vi "FPGA-code.vi"() -> ()   [LabVIEW 2020]
uses:
  <vilib>/Platform/TimedLoop/XDataNode/timing_clust.ctl
  <vilib>/Platform/TimedLoop/XDataNode/nitl_modes.ctl
  <vilib>/Platform/TimedLoop/XDataNode/wakeup.ctl
  <vilib>/rvi/IPIntegrationNode/IPINode_Typedef/niFpgaIPINodeSupportedFamilies.ctl
  <vilib>/rvi/Emulation/niFpgaGetClockAttributes.vi
  <vilib>/rvi/Emulation/niFpgaSctlEmulationGetInTimedLoop.vi
  <vilib>/rvi/Emulation/niFpgaEmulationReportErrorSimple.vi
  <vilib>/rvi/eio/common/nirviEmuTemplateMethod_errors.vi
  <vilib>/rvi/interface/RandomDataEmulation/nirviRandomDataMultiElementFPGAFIFO.vi
  <instcachedir>/0/nirviRandomDataMultiElementFPGAFIFO_3E9965BA1FAD4E7B8DABA31768A09B1F.lvgen/nirviRandomDataMultiElementFPGAFIFO_3E9965BA1FAD4E7B8DABA31768A09B1F_001.vi
  <vilib>/rvi/interface/RandomDataEmulation/niFpgaRandomDataHandleErrors.vi
  <vilib>/rvi/Emulation/niFpgaCriticalErrorInLSC.vi
  <instcachedir>/0/nirviRandomDataMultiElementFPGAFIFO_3E9965BA1FAD4E7B8DABA31768A09B1F.lvgen/nirviRandomDataMultiElementFPGAFIFO_3E9965BA1FAD4E7B8DABA31768A09B1F_000.vi
  <vilib>/rvi/IPIntegrationNode/IPINode_Utilities/niFpgaIPINodeSimCore.vi
  <vilib>/eio/EIONode/EIONode.xnode
  <vilib>/rvi/DataTransferAndStorage/Container/XNode/niFpgaContainer.xnode
  <vilib>/rvi/interface/RandomDataEmulation/nirviRandomDataFpgaMultiElementTemplate.vi
  <vilib>/rvi/interface/RandomDataEmulation/nirviRandomDataFpgaReadWriteTemplate.vi
  <vilib>/platform/TimedLoop/XDataNode/XDataNode.xnode
  <vilib>/rvi/IPIntegrationNode/IPINode_Xnode/niFpgaIPINode.xnode
  Simulink_ANN/hdl_prj/hdlsrc/ANN/IP_BlockSimFiles/xsim.dir/HDL_ANN/xsimk430938EFC64F42458762135EEBE48214.dll
  <vilib>/rvi/Memory/Memory_Emulation/nirvimemoryFastEmulation.vi
  <vilib>/rvi/Memory/Memory_Emulation/nirvimemoryEmulation.vi
  Global var FPGA.vi
  <vilib>/rvi/FIFO/Fifo_Resource/niFpgaFifoEmulationRefIn.vi
  <vilib>/Platform/TimedLoop/XDataNode/XDNodeRunTimeDep.lvlib
panel:
  out "Training Done":bool
  out "Inputs":bool[](array[boolean])
  out "Updated Weights and Biases":sgl[](array[numeric])
  out "2ndHiddenOut":sgl[](array[numeric])
  out "hidden 1":sgl[](array[numeric])
  out "Numeric":i32
  out "Data Read on iteration":i32
  out "Loop iteration":i32
  out "#Windows Handled":i16
  out "OutputLayerOut":sgl
  in  "Learning Rate":sgl=0.01
  in  "Data inputs":sgl=8.0
  out "Label expected output":sgl
  out "Initial Weigths and Biases":sgl[](array[numeric]) format="%.2f"
  out "Case Sleector":i16=3
  in  "stop":bool
  out "Array recived to multiply":sgl[](array[numeric])
  out "input Timed Out?":bool
  # "Node Values"
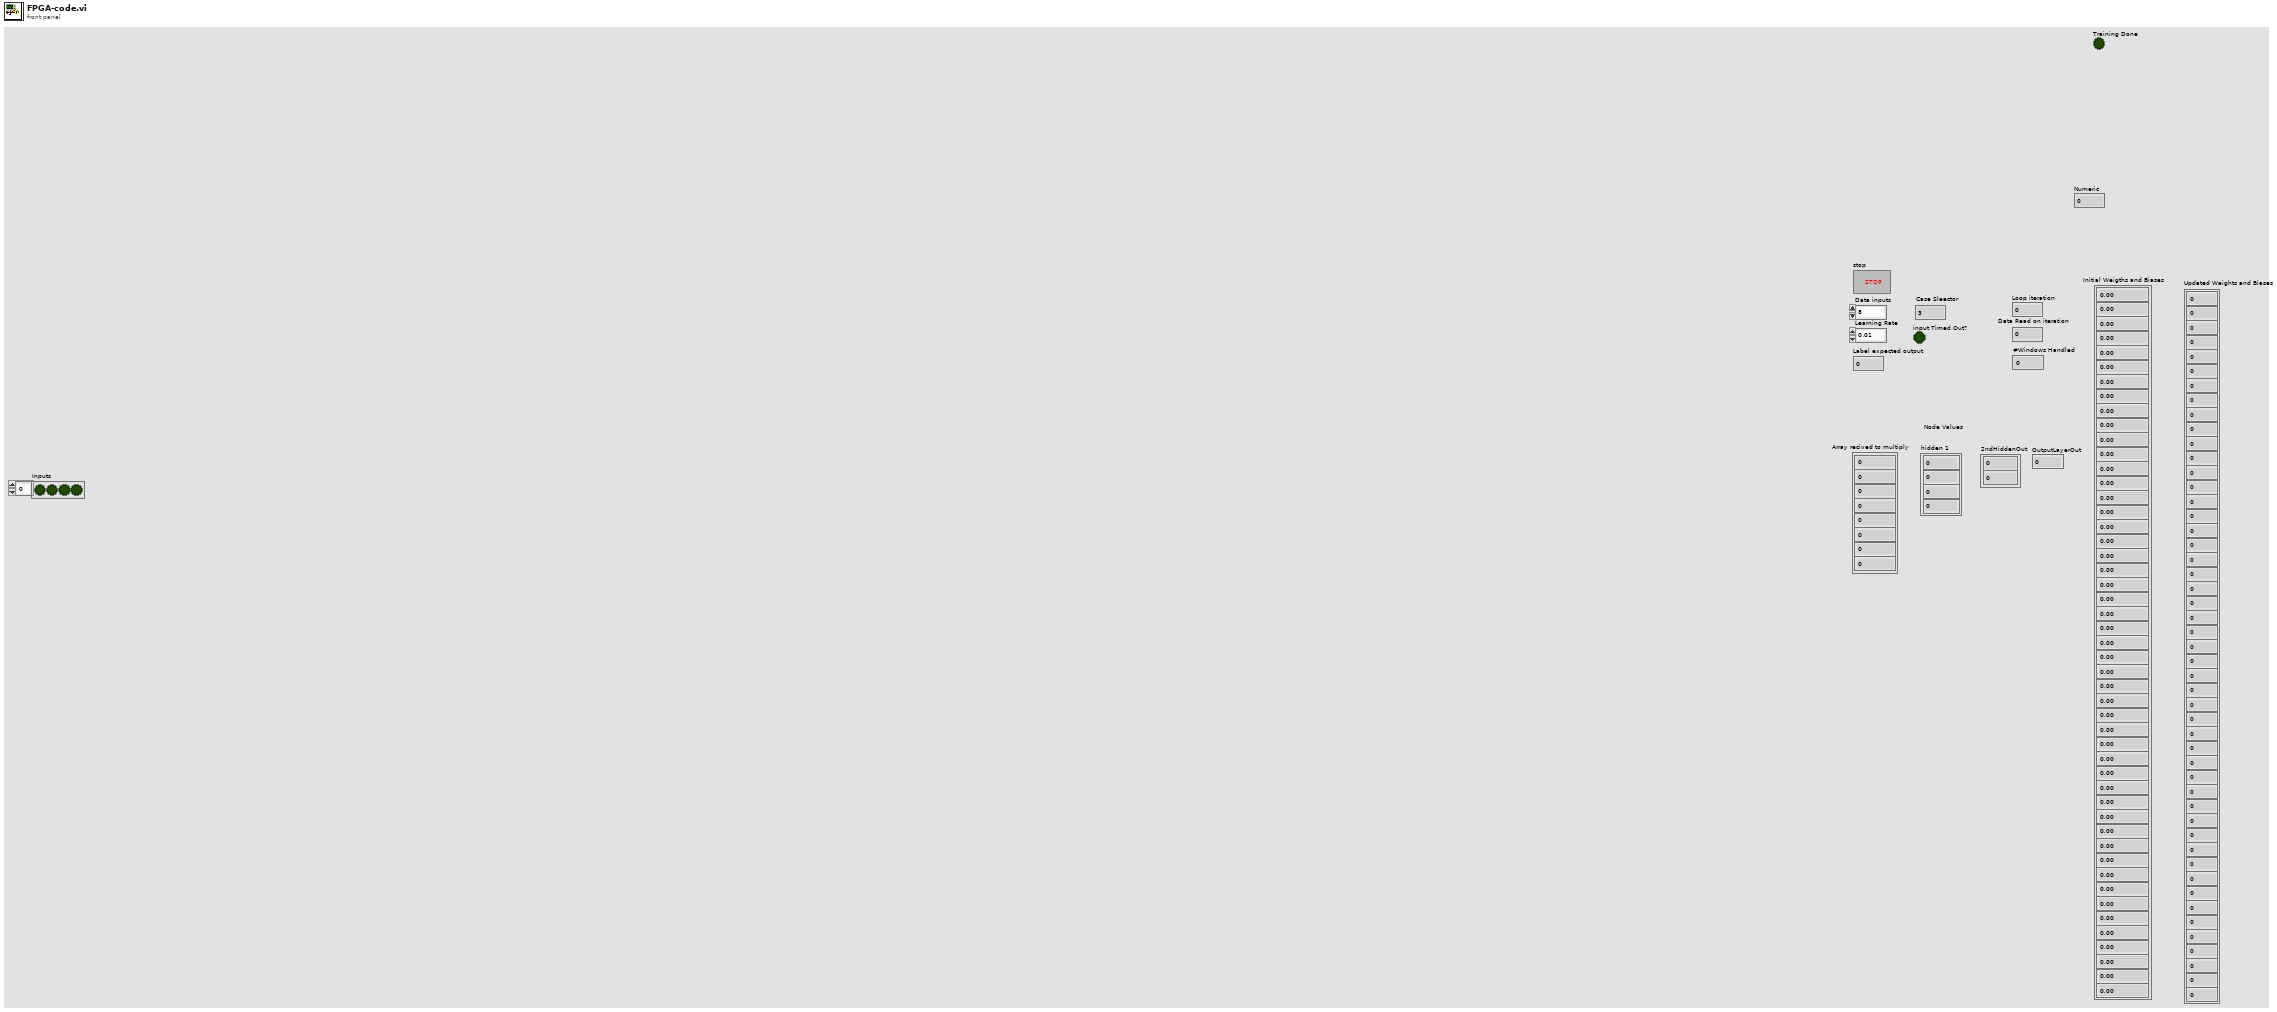
[diagram p1: front panel]
types:
  T1 = typedef "niFpgaIPINodeSupportedFamilies.ctl" = cluster{"unlimited?":bool, "supported targets":string[]}
  T2 = typedef "XDNodeRunTimeDep.lvlib/timing_clust.ctl" = cluster{"Expected End [f-1]":u64, "Actual End [f-1]":u64, "Finished Late? [f-1]":bool, "Expected End [i-1]":u64, "Actual End [i-1]":u64, "Finished Late? [i-1]":bool, "Expected Start [i]":u64, "Actual Start [i]":u64, "Expected Start [f]":u64, "Actual Start [f]":u64, "Source Name":string, "Structure Name":string, "Period":i64, "Deadline":i64, "Offset":i64, "Start":i64, "Priority":i32, "Timeout":i32, "Mode":T3, "Wakeup Reason":T4, "Error":errorcluster, "Source Type":string, "Secondary Source Type":string, "Global End Time":u64, "Global Start Time":u64, "Frame Duration":u64, "Iteration Duration":u64, "Assigned CPU":i32, "I/O Scan Engine Mode":u32}
  T3 = typedef "XDNodeRunTimeDep.lvlib/nitl_modes.ctl" = enum32{"No Change", "Process missed periods, maintain original phase", "Discard missed periods, maintain original phase", "Process missed periods, ignore original phase", "Discard missed periods, ignore original phase"}
  T4 = typedef "XDNodeRunTimeDep.lvlib/wakeup.ctl" = enum32{"Normal", "Aborted", "Asynchronous wakeup", "Timing source error", "Timed loop error", "Timeout"}
  T5 = cluster{"[0]":sgl, "[1]":sgl, "[2]":sgl, "[3]":sgl, "[4]":sgl, "[5]":sgl, "[6]":sgl, "[7]":sgl, "[8]":sgl, "[9]":sgl, "[10]":sgl, "[11]":sgl, "[12]":sgl, "[13]":sgl, "[14]":sgl, "[15]":sgl, "[16]":sgl, "[17]":sgl, "[18]":sgl, "[19]":sgl, "[20]":sgl, "[21]":sgl, "[22]":sgl, "[23]":sgl, "[24]":sgl}
  T6 = cluster{"Element[0]":sgl, "Element[1]":sgl, "Element[2]":sgl}
  T7 = cluster{sgl, sgl, sgl, sgl, sgl, sgl, sgl, sgl, sgl, sgl, sgl, sgl, sgl, sgl, sgl, sgl, sgl, sgl, sgl, sgl, sgl, sgl, sgl, sgl, sgl}
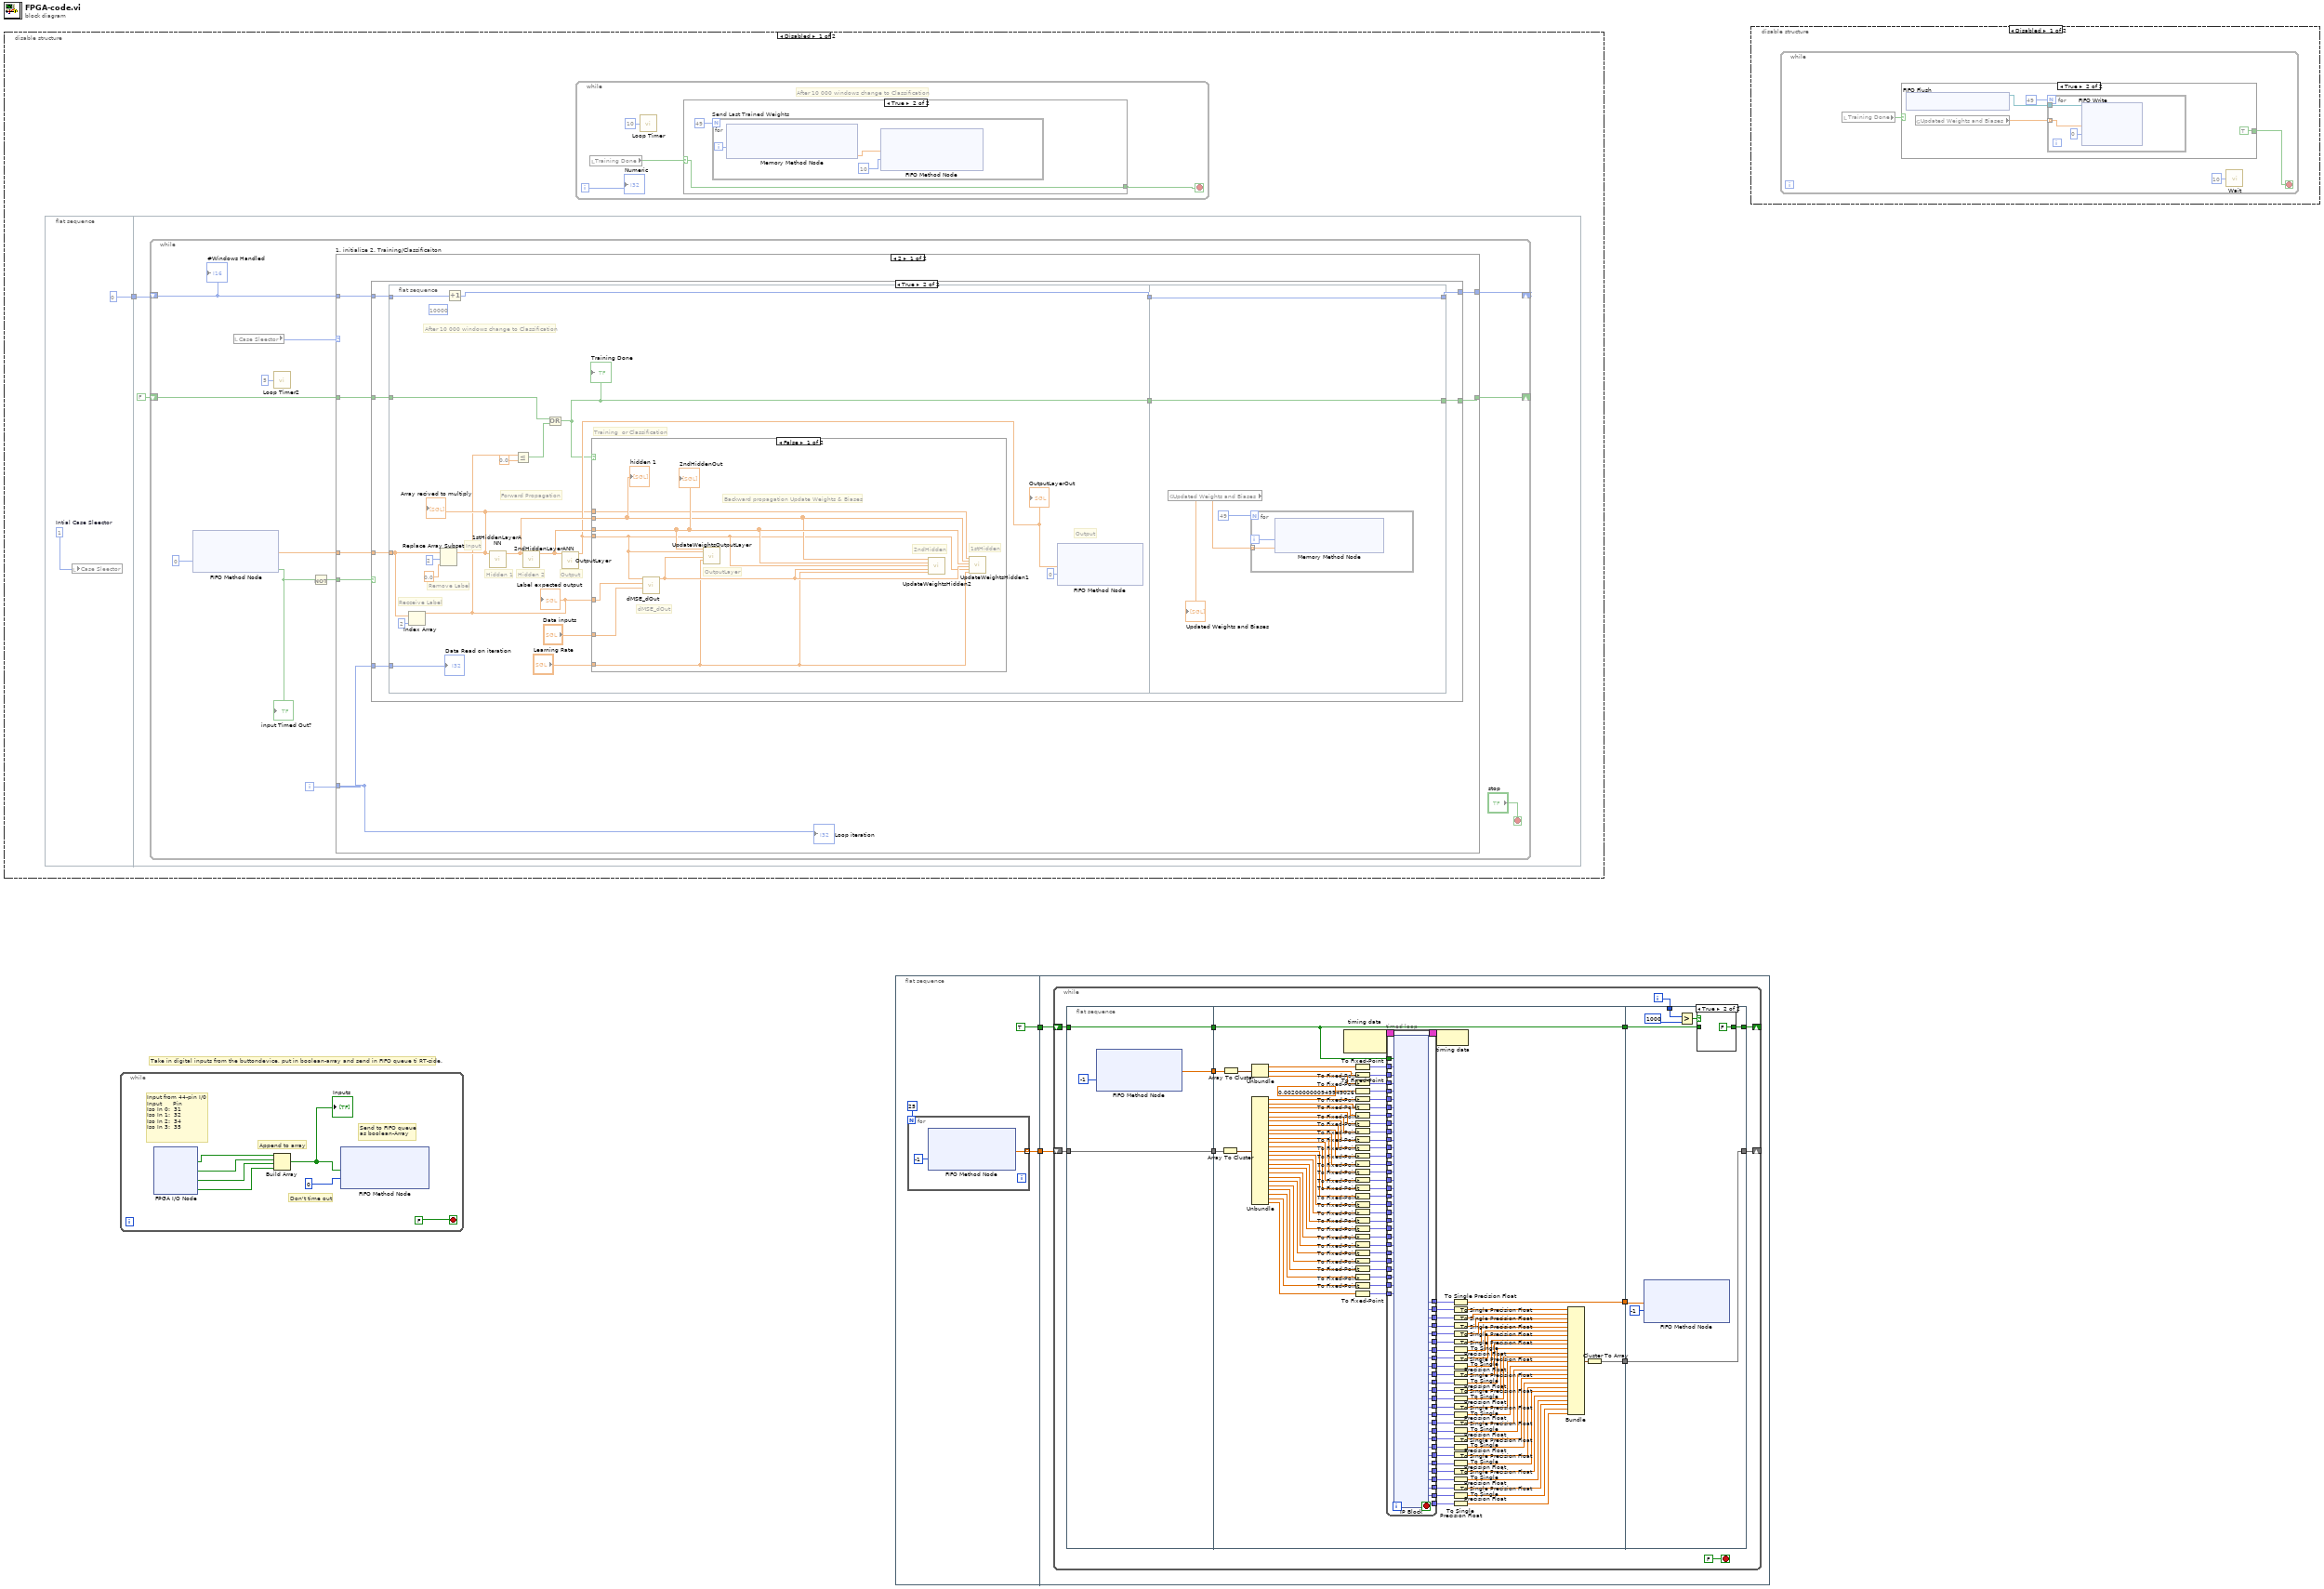
[diagram p0: block diagram]
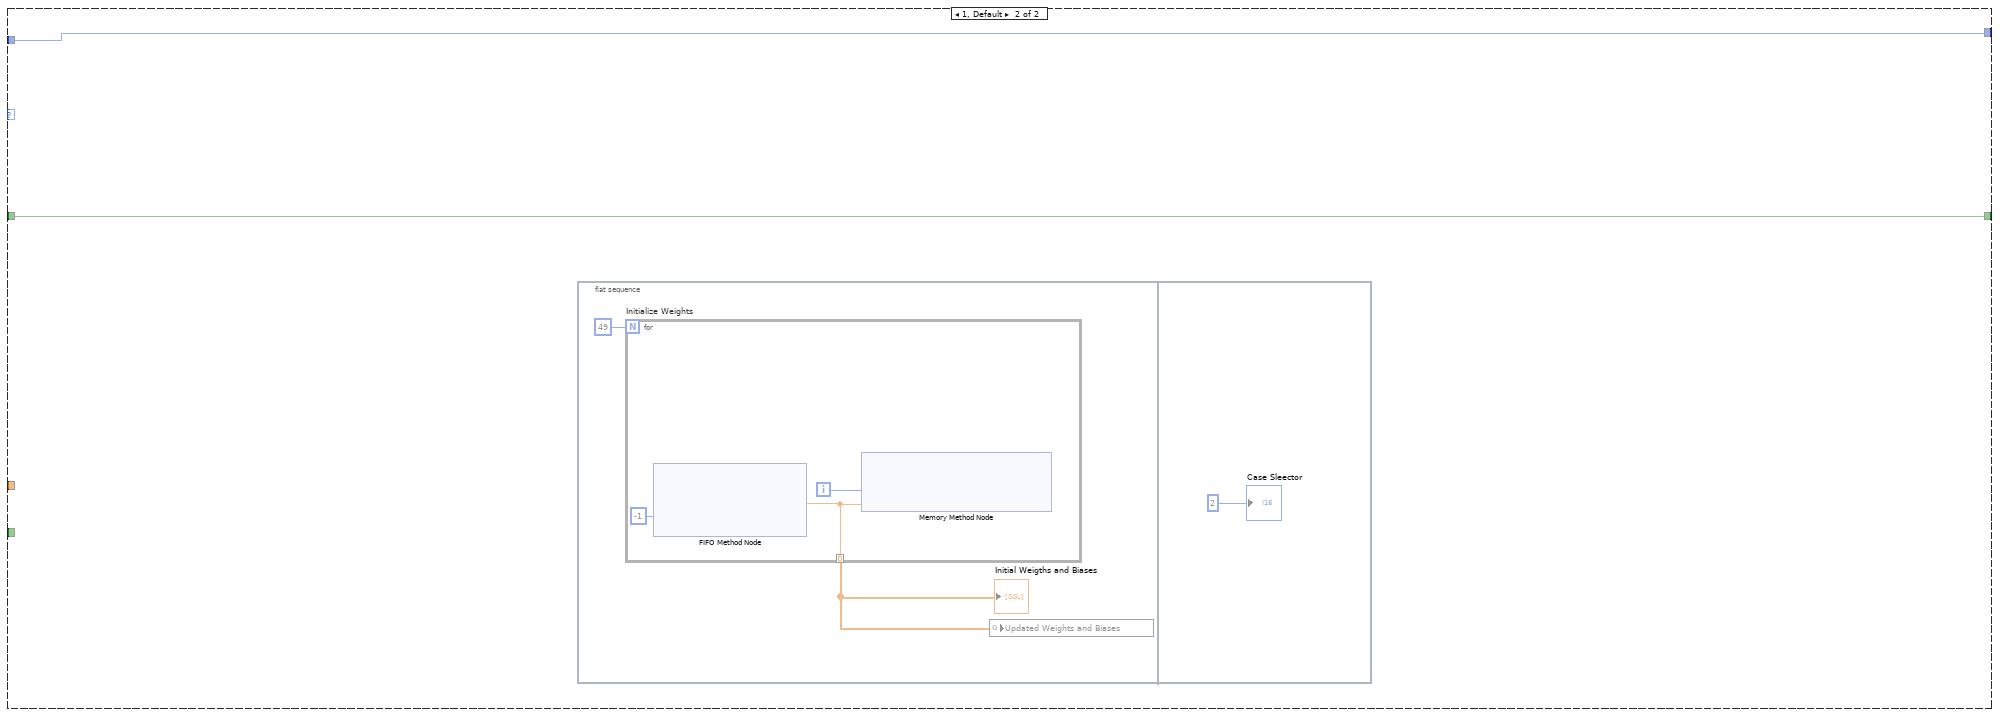
[diagram p5: hidden frame]
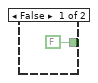
[diagram p8: hidden frame]
diagram:
  # "Take in digital inputs from the buttondevice, put in boolean-array and send in FIFO queue ti RT-side."
  n1 = disable-structure shown="Disabled" {
    frame Disabled {
      n2 = flat-sequence {
        tunnel: [i16 0] -> w3
        tunnel: w3 -> [w17]
        frame #0 {
          w15 = i16 1  # Intial Case Sleector
          n3 = local write "Case Sleector"(w15) -> ()
        }
        frame #1 {
          n4 = while {
            shift-right: [w24] -> _
            shift-left: w17 -> [w23]
            shift-right: [w18] -> _
            shift-left: FALSE -> [w19]
            i -> [w27]
            stop <- "stop" stop-if-true
            n5 = xnode ("FIFO Method Node")("Timeout"=0) -> ("Element"=w22:sgl[], "Timed Out?"=w26:bool)  [unwired: 2 in, 2 out]
            "input Timed Out?" <- w26
            n6 = local read "Case Sleector"() -> (w29:i16)
            n7 = call "Loop Timer2"("Count(mSec)"=u32 5) -> ()  [unwired: 1 out]
            n8 = Not(x=w26) -> (.not. x?=w25:bool)
            n9 = case "1. initialize 2. Training/Classificaiton" shown="2" w29 {
              tunnel: w27 -> [w35 _]
              tunnel: w25 -> [w36 _]
              tunnel: w23 -> [w34 w81]
              tunnel: [w33 w81] -> w24
              tunnel: w22 -> [w32 _]
              tunnel: w19 -> [w31 w80]
              tunnel: [w30 w80] -> w18
              frame 2 {
                n10 = case shown="True" w36 {
                  tunnel: w35 -> [_ w46]
                  tunnel: w34 -> [w38 w45]
                  tunnel: [w38 w44] -> w33
                  tunnel: w32 -> [_ w43]
                  tunnel: w31 -> [w37 w41]
                  tunnel: [w37 w39] -> w30
                  frame False {
                  }
                  frame True {
                    n11 = flat-sequence {
                      tunnel: w46 -> [w65]
                      tunnel: w45 -> [w64]
                      tunnel: w43 -> [w55]
                      tunnel: [w63] -> w42
                      tunnel: w41 -> [w47]
                      tunnel: [w49] -> w40
                      tunnel: [w77] -> w44
                      tunnel: w42 -> [w77]
                      tunnel: w40 -> [w75]
                      tunnel: [w75] -> w39
                      frame #0 {
                        (unwired) i16 10000 ("y")
                        # "Recceive Label"
                        # "Remove Label"
                        # "Training  or Classification"
                        # "After 10 000 windows change to Classification"
                        # "Output"
                        # "Output"
                        # "Hidden 2"
                        # "Hidden 1"
                        # "Input"
                        # "Forward Propagation"
                        n12 = Index Array(array=w55, index=2) -> (element=w51:sgl)
                        "Label expected output" <- w51
                        n13 = Replace Array Subset(array=w55, new element=sgl 0.0 ("new element/subarray"), index=2) -> (w53:sgl[])
                        "Array recived to multiply" <- w53
                        n14 = Increment(x=w64) -> (x+1=w63:i16)
                        n15 = call "1stHiddenLayerANN.vi"("Input"=w53) -> ("1stHiddenOut"=w61:sgl[])  [unwired: 10 in]
                        n16 = Less Or Equal?(x=w51, y=sgl 0.0) -> (x <= y?=w48:bool)
                        n17 = call "2ndHiddenLayerANN.vi"("2nd HiddenIn"=w61) -> ("2ndHiddenOut"=w59:sgl[])  [unwired: 9 in]
                        n18 = Or(x=w47, y=w48) -> (x .or. y?=w49:bool)
                        "Training Done" <- w49
                        n19 = call "OutputLayer.vi"("OutputlayerIn"=w59) -> ("OutputLayerOut"=w58:sgl)  [unwired: 14 in]
                        "OutputLayerOut" <- w58
                        n20 = case shown="False" w49 {
                          tunnel: "Data inputs" -> [w67 _]
                          tunnel: w61 -> [w70 _]
                          tunnel: "Learning Rate" -> [w72 _]
                          tunnel: w58 -> [w69 _]
                          tunnel: w59 -> [w71 _]
                          tunnel: w51 -> [w68 _]
                          tunnel: w53 -> [w66 _]
                          frame False {
                            # "1stHidden"
                            # "2ndHidden"
                            # "OutputLayer"
                            # "dMSE_dOut"
                            # "Backward propagation Update Weights & Biases"
                            n21 = call "dMSE_dOut.vi"("Data inputs"=w67, "Label (expected output"=w68, "Output"=w69) -> ("Numeric"=w73:sgl)  [unwired: 8 in]
                            n22 = call "UpdateWeightsOutputLayer.vi"("OutputH2"=w71, "Final Output"=w69, "dEtot_dOut"=w73, "Learning Rate"=w72) -> ()  [unwired: 16 in]
                            n23 = call "UpdateWeightsHidden2.vi"("OutH1"=w70, "OutH2"=w71, "Output"=w69, "dEtot_dOut"=w73, "Learning Rate"=w72) -> ()  [unwired: 11 in]
                            n24 = call "UpdateWeightsHidden1.vi"("Input"=w66, "OutH1"=w70, "OutH2"=w71, "dEOut_dOut"=w73, "Output"=w69, "Learning Rate"=w72) -> ()  [unwired: 14 in]
                            "hidden 1" <- w70
                            "2ndHiddenOut" <- w71
                          }
                          frame True {
                          }
                        }
                        n25 = xnode ("FIFO Method Node")("Element"=w58, "Timeout"=0) -> ()  [unwired: 1 in, 2 out]
                        "Data Read on iteration" <- w65
                      }
                      frame #1 {
                        n26 = global read "Global var FPGA.vi" "Updated Weights and Biases"() -> (w76:sgl[])
                        "Updated Weights and Biases" <- w76
                        n27 = for "Send Last Trained Weights" {
                          N: 49 -> [_]
                          tunnel: w76 -> [w78] mode=indexing
                          i -> [w79]
                          n28 = xnode ("Memory Method Node")("Address"=w79, "Data"=w78) -> ()  [unwired: 1 in, 1 out]
                        }
                      }
                    }
                  }
                }
                "Loop iteration" <- w35
              }
              frame 1, Default {
                n29 = flat-sequence {
                  frame #0 {
                    n30 = for "Initialize Weights" {
                      N: 49 -> [_]
                      tunnel: [w84] -> w82 mode=indexing
                      i -> [w86]
                      n31 = xnode ("FIFO Method Node")("Timeout"=-1) -> ("Element"=w84:sgl)  [unwired: 1 in, 2 out]
                      n32 = xnode ("Memory Method Node")("Address"=w86, "Data"=w84) -> ()  [unwired: 1 in, 1 out]
                    }
                    "Initial Weigths and Biases" <- w82
                    n33 = global write "Global var FPGA.vi" "Updated Weights and Biases"(w82) -> ()
                  }
                  frame #1 {
                    "Case Sleector" <- i16 2 ("Numeric 3")
                  }
                }
              }
            }
            "#Windows Handled" <- w23
          }
        }
      }
      n34 = while {
        i -> [w5]
        stop <- w6 stop-if-true
        # "After 10 000 windows change to Classification"
        n35 = local read "Training Done"() -> (w7:bool)
        n36 = call "Loop Timer"("Count(mSec)"=u32 10) -> ()  [unwired: 1 out]
        n37 = case shown="True" w7 {
          selector: w7 -> [w8 w9]
          tunnel: [w8 w9] -> w6
          frame False {
          }
          frame True {
            n38 = for "Send Last Trained Weights" {
              N: 49 -> [_]
              i -> [w13]
              n39 = xnode ("Memory Method Node")("Address"=w13) -> ("Data"=w12:sgl)  [unwired: 1 in, 1 out]
              n40 = xnode ("FIFO Method Node")("Element"=w12, "Timeout"=10) -> ()  [unwired: 1 in, 2 out]
            }
          }
        }
        "Numeric" <- w5
      }
    }
    frame Enabled {
    }
  }
  n41 = while {
    stop <- FALSE stop-if-true
    # "Don't time out"
    # "Append to array"
    # "Send to FIFO queue\nas boolean-Array"
    # "Input from 44-pin I/0\nInput      Pin\nIso In 0:  31\nIso In 1:  32\nIso In 2:  34\nIso In 3:  35"
    n42 = xnode "FPGA I/O Node"() -> ("Iso In 0"=w93:bool, "Iso In 1"=w90:bool, "Iso In 2"=w89:bool, "Iso In 3"=w88:bool)  [unwired: 4 in, 4 out]
    n43 = Build Array(w93, w90, w89, w88) -> (w91:bool[])
    "Inputs" <- w91
    n44 = xnode ("FIFO Method Node")("Element"=w91, "Timeout"=0) -> ()  [unwired: 1 in, 2 out]
  }
  n45 = flat-sequence {
    tunnel: [w96] -> w2
    tunnel: [TRUE] -> w1
    tunnel: w2 -> [w101]
    tunnel: w1 -> [w100]
    frame #0 {
      n46 = for {
        N: 25 -> [_]
        tunnel: [w98] -> w96 mode=indexing
        n47 = xnode ("FIFO Method Node")("Timeout"=-1) -> ("Element"=w98:sgl)  [unwired: 1 in, 2 out]
      }
    }
    frame #1 {
      n48 = while {
        shift-right: [w109] -> _
        shift-left: w101 -> [w108]
        shift-right: [w106] -> _
        shift-left: w100 -> [w103]
        i -> [w102]
        stop <- FALSE stop-if-true
        n49 = flat-sequence {
          tunnel: [w115] -> w113
          tunnel: [w116] -> w112
          tunnel: w108 -> [w115]
          tunnel: [w114] -> w104
          tunnel: w103 -> [w114]
          tunnel: w113 -> [w130]
          tunnel: w112 -> [w212]
          tunnel: [w127] -> w110
          tunnel: [w125] -> w107
          tunnel: [w120] -> w105
          tunnel: w104 -> [w120]
          tunnel: w110 -> [w561]
          tunnel: [w561] -> w109
          tunnel: w107 -> [w560]
          tunnel: [w559] -> w106
          tunnel: w105 -> [w558]
          tunnel: w102 -> [w556]
          frame #0 {
            n50 = xnode ("FIFO Method Node")("Timeout"=-1) -> ("Element"=w116:sgl[])  [unwired: 2 in, 3 out]
          }
          frame #1 {
            n51 = Array To Cluster(array=w130) -> (cluster=w180:T5)
            n52 = Array To Cluster(array=w212) -> (cluster=w211:T6)
            n53 = Unbundle(w211) -> ("Element[0]"=w210:sgl, "Element[1]"=w209:sgl, "Element[2]"=w123:sgl)
            n54 = Unbundle(w180) -> ("[0]"=w208:sgl, "[1]"=w236:sgl, "[2]"=w235:sgl, "[3]"=w234:sgl, "[4]"=w233:sgl, "[5]"=w232:sgl, "[6]"=w231:sgl, "[7]"=w230:sgl, "[8]"=w229:sgl, "[9]"=w228:sgl, "[10]"=w227:sgl, "[11]"=w226:sgl, "[12]"=w225:sgl, "[13]"=w224:sgl, "[14]"=w223:sgl, "[15]"=w222:sgl, "[16]"=w221:sgl, "[17]"=w220:sgl, "[18]"=w219:sgl, "[19]"=w218:sgl, "[20]"=w217:sgl, "[21]"=w216:sgl, "[22]"=w215:sgl, "[23]"=w214:sgl, "[24]"=w213:sgl)
            n55 = node-c288() -> (w119:T2)  [unwired: 1 in]
            n56 = To Fixed-Point(number=w210) -> (fixed-point=w207:fxp<+/-,18,12>)  [unwired: 1 in]
            n57 = To Fixed-Point(number=w209) -> (fixed-point=w206:fxp<+/-,18,12>)  [unwired: 1 in]
            n58 = To Fixed-Point(number=w123) -> (fixed-point=w124:fxp<+/-,18,12>)  [unwired: 1 in]
            n59 = To Fixed-Point(number=sgl 0.002) -> (fixed-point=w122:fxp<+/-,18,12>)  [unwired: 1 in]
            n60 = To Fixed-Point(number=w208) -> (fixed-point=w205:fxp<+/-,18,12>)  [unwired: 1 in]
            n61 = To Fixed-Point(number=w236) -> (fixed-point=w204:fxp<+/-,18,12>)  [unwired: 1 in]
            n62 = To Fixed-Point(number=w235) -> (fixed-point=w203:fxp<+/-,18,12>)  [unwired: 1 in]
            n63 = To Fixed-Point(number=w234) -> (fixed-point=w202:fxp<+/-,18,12>)  [unwired: 1 in]
            n64 = To Fixed-Point(number=w233) -> (fixed-point=w201:fxp<+/-,18,12>)  [unwired: 1 in]
            n65 = To Fixed-Point(number=w232) -> (fixed-point=w200:fxp<+/-,18,12>)  [unwired: 1 in]
            n66 = To Fixed-Point(number=w231) -> (fixed-point=w199:fxp<+/-,18,12>)  [unwired: 1 in]
            n67 = To Fixed-Point(number=w230) -> (fixed-point=w198:fxp<+/-,18,12>)  [unwired: 1 in]
            n68 = To Fixed-Point(number=w229) -> (fixed-point=w197:fxp<+/-,18,12>)  [unwired: 1 in]
            n69 = To Fixed-Point(number=w228) -> (fixed-point=w196:fxp<+/-,18,12>)  [unwired: 1 in]
            n70 = To Fixed-Point(number=w227) -> (fixed-point=w195:fxp<+/-,18,12>)  [unwired: 1 in]
            n71 = To Fixed-Point(number=w226) -> (fixed-point=w194:fxp<+/-,18,12>)  [unwired: 1 in]
            n72 = To Fixed-Point(number=w225) -> (fixed-point=w193:fxp<+/-,18,12>)  [unwired: 1 in]
            n73 = To Fixed-Point(number=w224) -> (fixed-point=w192:fxp<+/-,18,12>)  [unwired: 1 in]
            n74 = To Fixed-Point(number=w223) -> (fixed-point=w191:fxp<+/-,18,12>)  [unwired: 1 in]
            n75 = To Fixed-Point(number=w222) -> (fixed-point=w190:fxp<+/-,18,12>)  [unwired: 1 in]
            n76 = To Fixed-Point(number=w221) -> (fixed-point=w189:fxp<+/-,18,12>)  [unwired: 1 in]
            n77 = To Fixed-Point(number=w220) -> (fixed-point=w188:fxp<+/-,18,12>)  [unwired: 1 in]
            n78 = To Fixed-Point(number=w219) -> (fixed-point=w187:fxp<+/-,18,12>)  [unwired: 1 in]
            n79 = To Fixed-Point(number=w218) -> (fixed-point=w186:fxp<+/-,18,12>)  [unwired: 1 in]
            n80 = To Fixed-Point(number=w217) -> (fixed-point=w185:fxp<+/-,18,12>)  [unwired: 1 in]
            n81 = To Fixed-Point(number=w216) -> (fixed-point=w184:fxp<+/-,18,12>)  [unwired: 1 in]
            n82 = To Fixed-Point(number=w215) -> (fixed-point=w183:fxp<+/-,18,12>)  [unwired: 1 in]
            n83 = To Fixed-Point(number=w214) -> (fixed-point=w182:fxp<+/-,18,12>)  [unwired: 1 in]
            n84 = To Fixed-Point(number=w213) -> (fixed-point=w181:fxp<+/-,18,12>)  [unwired: 1 in]
            n85 = timed-loop {
              timing: w119 -> [_]
              timing-out: [_] -> w118
              tunnel: w207 -> [w292]
              tunnel: w206 -> [w291]
              tunnel: w205 -> [w290]
              tunnel: w204 -> [w289]
              tunnel: w203 -> [w288]
              tunnel: w202 -> [w287]
              tunnel: w201 -> [w286]
              tunnel: w200 -> [w285]
              tunnel: w199 -> [w284]
              tunnel: w198 -> [w283]
              tunnel: w197 -> [w282]
              tunnel: w196 -> [w281]
              tunnel: w195 -> [w280]
              tunnel: w194 -> [w279]
              tunnel: w193 -> [w278]
              tunnel: w192 -> [w277]
              tunnel: w191 -> [w276]
              tunnel: w190 -> [w275]
              tunnel: w189 -> [w274]
              tunnel: w188 -> [w273]
              tunnel: w187 -> [w272]
              tunnel: w186 -> [w271]
              tunnel: w185 -> [w270]
              tunnel: w184 -> [w269]
              tunnel: w183 -> [w268]
              tunnel: w182 -> [w267]
              tunnel: w181 -> [w266]
              tunnel: [w265] -> w179
              tunnel: [w264] -> w178
              tunnel: [w263] -> w177
              tunnel: [w262] -> w176
              tunnel: [w261] -> w175
              tunnel: [w260] -> w174
              tunnel: [w259] -> w173
              tunnel: [w258] -> w172
              tunnel: [w257] -> w171
              tunnel: [w256] -> w170
              tunnel: [w255] -> w169
              tunnel: [w254] -> w168
              tunnel: [w253] -> w167
              tunnel: [w252] -> w166
              tunnel: [w251] -> w165
              tunnel: [w250] -> w164
              tunnel: [w249] -> w163
              tunnel: [w248] -> w162
              tunnel: [w247] -> w161
              tunnel: [w246] -> w160
              tunnel: [w245] -> w159
              tunnel: [w244] -> w158
              tunnel: [w243] -> w157
              tunnel: [w242] -> w156
              tunnel: [w241] -> w147
              tunnel: [w240] -> w126
              tunnel: w124 -> [w239]
              tunnel: w122 -> [w238]
              tunnel: w120 -> [w237]
              stop <- _ stop-if-true
              n86 = xnode ("IP Block")("train_1"=w237, "input_0"=w292, "input_1"=w291, "target"=w239, "alpha"=w238, "w1_0"=w290, "w1_1"=w289, "w1_2"=w288, "w1_3"=w287, "w1_4"=w286, "w1_5"=w285, "w1_6"=w284, "w1_7"=w283, "w2_0"=w282, "w2_1"=w281, "w2_2"=w280, "w2_3"=w279, "w2_4"=w278, "w2_5"=w277, "w2_6"=w276, "w2_7"=w275, "w3_0"=w274, "w3_1"=w273, "b1_0"=w272, "b1_1"=w271, "b1_2"=w270, "b1_3"=w269, "b2_0"=w268, "b2_1"=w267, "b3"=w266) -> ("output"=w240:fxp<+/-,18,12>, "w1_out_0"=w265:fxp<+/-,18,12>, "w1_out_1"=w263:fxp<+/-,18,12>, "w1_out_2"=w262:fxp<+/-,18,12>, "w1_out_3"=w261:fxp<+/-,18,12>, "w1_out_4"=w260:fxp<+/-,18,12>, "w1_out_5"=w259:fxp<+/-,18,12>, "w1_out_6"=w258:fxp<+/-,18,12>, "w1_out_7"=w257:fxp<+/-,18,12>, "w2_out_0"=w256:fxp<+/-,18,12>, "w2_out_1"=w250:fxp<+/-,18,12>, "w2_out_2"=w251:fxp<+/-,18,12>, "w2_out_3"=w252:fxp<+/-,18,12>, "w2_out_4"=w253:fxp<+/-,18,12>, "w2_out_5"=w249:fxp<+/-,18,12>, "w2_out_6"=w248:fxp<+/-,18,12>, "w2_out_7"=w247:fxp<+/-,18,12>, "w3_out_0"=w254:fxp<+/-,18,12>, "w3_out_1"=w246:fxp<+/-,18,12>, "b1_out_0"=w245:fxp<+/-,18,12>, "b1_out_1"=w244:fxp<+/-,18,12>, "b1_out_2"=w243:fxp<+/-,18,12>, "b1_out_3"=w242:fxp<+/-,18,12>, "b2_out_0"=w255:fxp<+/-,18,12>, "b2_out_1"=w264:fxp<+/-,18,12>, "b3_out"=w241:fxp<+/-,18,12>)
            }
            n87 = node-c288(w118) -> ()
            n88 = To Single Precision Float(number=w126) -> (single precision float=w125:sgl)
            n89 = To Single Precision Float(number=w179) -> (single precision float=w129:sgl)
            n90 = To Single Precision Float(number=w177) -> (single precision float=w155:sgl)
            n91 = To Single Precision Float(number=w176) -> (single precision float=w154:sgl)
            n92 = To Single Precision Float(number=w175) -> (single precision float=w153:sgl)
            n93 = To Single Precision Float(number=w174) -> (single precision float=w152:sgl)
            n94 = To Single Precision Float(number=w173) -> (single precision float=w151:sgl)
            n95 = To Single Precision Float(number=w172) -> (single precision float=w150:sgl)
            n96 = To Single Precision Float(number=w171) -> (single precision float=w149:sgl)
            n97 = To Single Precision Float(number=w170) -> (single precision float=w148:sgl)
            n98 = To Single Precision Float(number=w164) -> (single precision float=w146:sgl)
            n99 = To Single Precision Float(number=w165) -> (single precision float=w145:sgl)
            n100 = To Single Precision Float(number=w166) -> (single precision float=w144:sgl)
            n101 = To Single Precision Float(number=w167) -> (single precision float=w143:sgl)
            n102 = To Single Precision Float(number=w163) -> (single precision float=w142:sgl)
            n103 = To Single Precision Float(number=w162) -> (single precision float=w141:sgl)
            n104 = To Single Precision Float(number=w161) -> (single precision float=w140:sgl)
            n105 = To Single Precision Float(number=w168) -> (single precision float=w139:sgl)
            n106 = To Single Precision Float(number=w160) -> (single precision float=w138:sgl)
            n107 = To Single Precision Float(number=w159) -> (single precision float=w137:sgl)
            n108 = To Single Precision Float(number=w158) -> (single precision float=w136:sgl)
            n109 = To Single Precision Float(number=w157) -> (single precision float=w135:sgl)
            n110 = To Single Precision Float(number=w156) -> (single precision float=w134:sgl)
            n111 = To Single Precision Float(number=w169) -> (single precision float=w133:sgl)
            n112 = To Single Precision Float(number=w178) -> (single precision float=w132:sgl)
            n113 = To Single Precision Float(number=w147) -> (single precision float=w131:sgl)
            n114 = Bundle(w129, w155, w154, w153, w152, w151, w150, w149, w148, w146, w145, w144, w143, w142, w141, w140, w139, w138, w137, w136, w135, w134, w133, w132, w131) -> (w128:T7)  [unwired: 1 in]
            n115 = Cluster To Array(cluster=w128) -> (array=w127:sgl[])
          }
          frame #2 {
            n116 = xnode ("FIFO Method Node")("Element"=w560, "Timeout"=-1) -> ()  [unwired: 1 in, 2 out]
            n117 = Greater?(x=w556, y=i16 1000) -> (0:w555:bool)
            n118 = case shown="True" w555 {
              tunnel: [w562 FALSE] -> w559
              tunnel: w558 -> [w562 _]
              frame False {
              }
              frame True {
              }
            }
          }
        }
      }
    }
  }
  n119 = disable-structure shown="Disabled" {
    frame Disabled {
      n120 = while {
        stop <- w564 stop-if-true
        n121 = local read "Training Done"() -> (w565:bool)
        n122 = case shown="True" w565 {
          tunnel: [FALSE TRUE] -> w564
          frame False {
          }
          frame True {
            n123 = xnode ("FIFO Flush")() -> ("FIFO Out"=w569:refnum<k21>)  [unwired: 1 in]
            n124 = global read "Global var FPGA.vi" "Updated Weights and Biases"() -> (w571:sgl[])
            n125 = for {
              N: 49 -> [_]
              tunnel: w571 -> [w574] mode=indexing
              tunnel: w569 -> [w572]
              n126 = xnode ("FIFO Write")("Element"=w574, "Timeout"=0, "FIFO In"=w572) -> ()  [unwired: 2 out]
            }
          }
        }
        n127 = call "Wait"("Count(Ticks)"=u32 10) -> ()  [unwired: 1 out]
      }
    }
    frame Enabled {
    }
  }
